vi "Create Serializer VI.vi"(0 "VI in":refnum<vi>, 11 "error in (no error)":errorcluster) -> (4 "SubVI out":refnum<vi>, 15 "error out":errorcluster)   [LabVIEW 2021, in "Migrator.lvlib"]
uses:
  Migrator.lvlib
  <vilib>/Utility/miscctls.llb/LVPointTypeDef.ctl
  Path Functions/Path Functions.lvlib
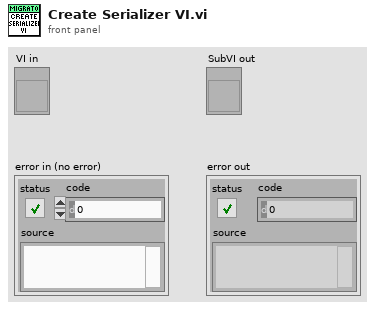
[diagram p1: front panel]
types:
  T1 = typedef "LVPointTypeDef.ctl" = cluster{"Horizontal":i16, "Vertical":i16}
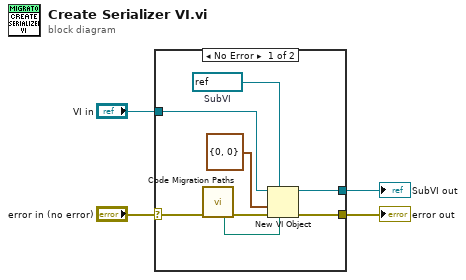
[diagram p0: block diagram]
diagram:
  n1 = case shown="No Error" "error in (no error)" {
    selector: "error in (no error)" -> [w12 w13]
    tunnel: [w10 w13] -> w3
    tunnel: [w9 _] -> w2
    tunnel: "VI in" -> [w8 _]
    frame No Error {
      w5 = refnum<vi> refnum  # SubVI
      n2 = call "Code Migration Paths.vi"("error in (no error)"=w12) -> ("Serializer"=w6:path, "error out"=w7:errorcluster)  [unwired: 6 in, 7 out]
      n3 = New VI Object(vi object class=w5, owner refnum=w8, position/next to=T1 {"Horizontal"=0, "Vertical"=0} ("location"), 6:w6, 8:w7) -> (object refnum=w9:refnum<vi>, 0:w10:errorcluster)  [unwired: 3 in]
    }
    frame Error {
    }
  }
  "error out" <- w3
  "SubVI out" <- w2
